vi "Reconstitute LQIdentity.vi"(8 "Error In":errorcluster, 10 "Manifestation":u64, 11 "LQIdentity Prototype":refnum<class "LQIdentity.lvclass">) -> (0 "Error Out":errorcluster, 3 "Reconstituted LQIdentity":refnum<class "LQIdentity.lvclass">)   [LabVIEW 2013, in "Template.lvlib" / "LQWidgetEngine.lvclass"]
uses:
  LQWidgetEngine.lvclass
  LQIdentity/LQIdentity.lvclass
  LQIdentity Registry Action.ctl
  LQIdentity/LQIdentity.lvclass/LQIdentity.ctl
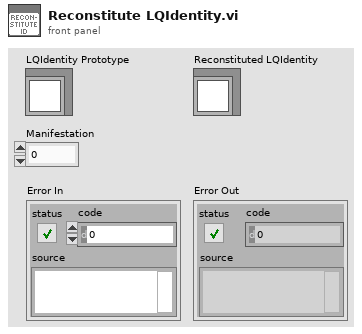
[diagram p1: front panel]
types:
  T1 = typedef "Template.lvlib/LQWidgetEngine.lvclass/LQIdentity Registry Action.ctl" = enum16{"Init", "Register LQIdentity", "Get LQIdentity Info", "Deregister LQIdentity"}
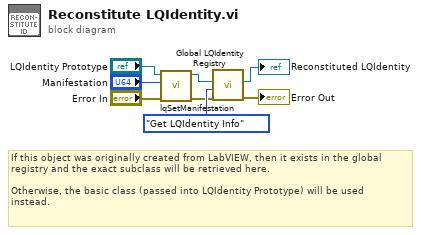
[diagram p0: block diagram]
diagram:
  # "If this object was originally created from LabVIEW, then it exists in the global\nregistry and the exact subclass will be retrieved here.\n\nOtherwise, the basic class (passed into LQIdentity Prototype) will be used\ninstead."
  n1 = call "lqSetManifestation.vi"("Error In"="Error In", "Manifestation"="Manifestation", "LQIdentity in"="LQIdentity Prototype") -> ("Error Out"=w3:errorcluster, "LQIdentity out"=w5:refnum<class "LQIdentity.lvclass">)  [unwired: 7 in]
  n2 = call "Global LQIdentity Registry.vi"("Error In"=w3, "Registry Action"=LQIdentity_Registry_Action."Get LQIdentity Info" ("LQIdentity Registry Action"), "LQIdentity Info In"=w5) -> ("Error Out"=→"Error Out":errorcluster, "LQIdentity Info Out"=→"Reconstituted LQIdentity":refnum<class "LQIdentity.lvclass">)  [unwired: 7 in]
